vi "SetConfiguredPieceObj.vi"(8 "error in (no error)":errorcluster, 10 "configuredPieceObj":refnum<class "Piece.lvclass">, 11 "object in":refnum<class "Board.lvclass">) -> (0 "error out":errorcluster, 3 "object out":refnum<class "Board.lvclass">)   [LabVIEW 2020, in "Board.lvclass"]
uses:
  Board.lvclass
  Pieces/Piece.lvclass
  Board.lvclass/Board.ctl
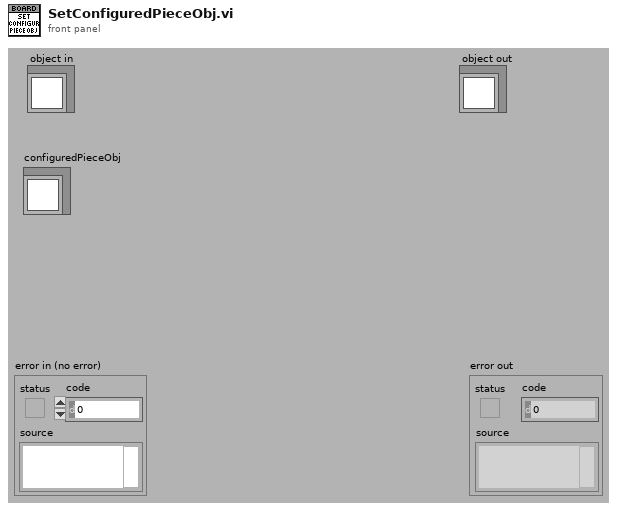
[diagram p1: front panel]
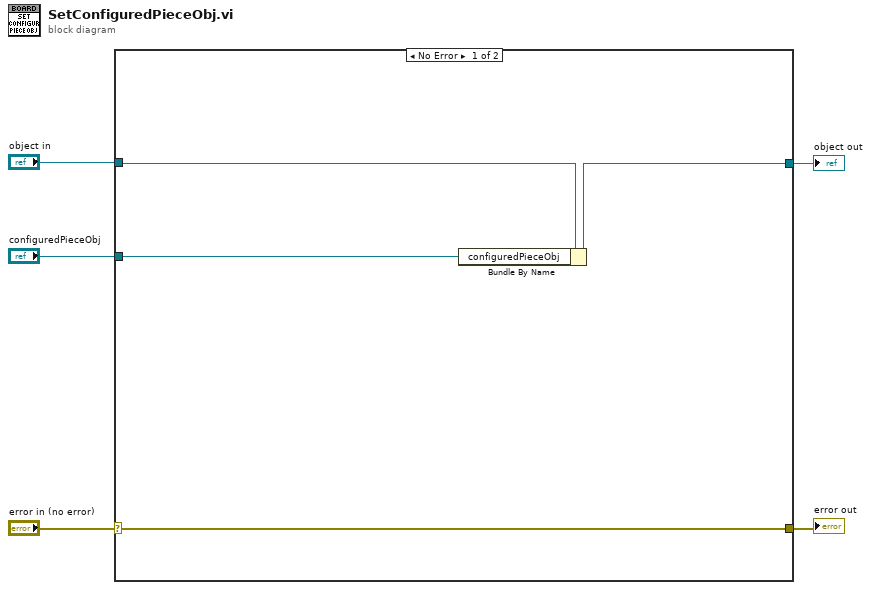
[diagram p0: block diagram]
diagram:
  n1 = case shown="No Error" "error in (no error)" {
    selector: "error in (no error)" -> [w8 w11]
    tunnel: [w8 w11] -> w4
    tunnel: [w6 w10] -> w2
    tunnel: "object in" -> [w7 w10]
    tunnel: "configuredPieceObj" -> [w9 _]
    frame No Error {
      n2 = Bundle By Name(cluster=w7, "configuredPieceObj"=w9) -> (w6:refnum<class "Board.lvclass">)
    }
    frame Error {
    }
  }
  "error out" <- w4
  "object out" <- w2
